vi "PRIME Telescope Convert HHMMSS string.vi"(10 "RA String":string) -> (1 "Array":dbl[](array[numeric]), 2 "Right Ascension":T1)   [LabVIEW 2024, in "PRIME Telescope.lvclass"]
uses:
  PRIME Telescope.lvclass
  library/lib cluster HH MM SEC.ctl
  <vilib>/regexp/Match Regular Expression.xnode
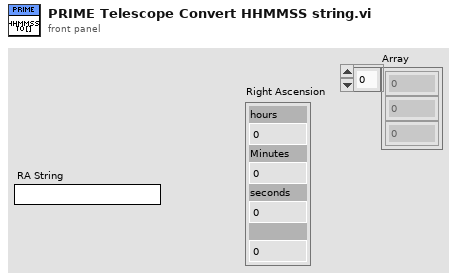
[diagram p1: front panel]
types:
  T1 = typedef "lib cluster HH MM SEC.ctl" = cluster{"hours":dbl, "Minutes":dbl, "seconds":dbl, "sign":dbl}
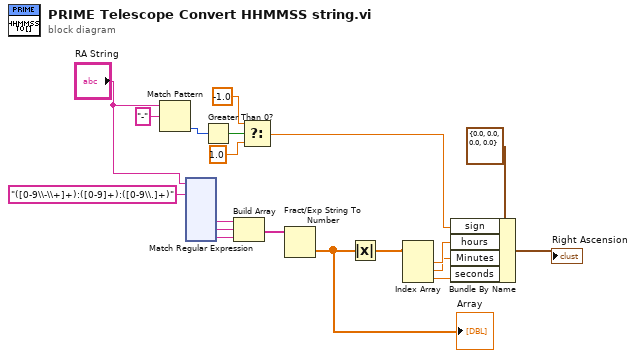
[diagram p0: block diagram]
diagram:
  n1 = Match Pattern(string="RA String", regular expression="-") -> (offset past match=w12:i32)  [unwired: 1 in, 3 out]
  n2 = xnode "Match Regular Expression"("input string"="RA String", "regular expression"="([0-9\\-\\+]+):([0-9]+):([0-9\\.]+)") -> ("submatch 1"=w18:string, "submatch 2"=w17:string, "submatch 3"=w16:string)  [unwired: 4 in, 5 out]
  n3 = Greater Than 0?(x=w12) -> (x > 0?=w4:bool)
  n4 = Build Array(w18, w17, w16) -> (w15:string[])
  n5 = Select(t=-1.0, s=w4, f=1.0) -> (s? t:f=w3:dbl)
  n6 = Fract/Exp String To Number(string=w15) -> (number=w11:dbl[])  [unwired: 3 in, 1 out]
  "Array" <- w11
  n7 = Absolute Value(x=w11) -> (abs(x)=w9:dbl[])
  n8 = Index Array(array=w9) -> (element #1=w8:dbl, element #2=w7:dbl, element #3=w6:dbl)  [unwired: 3 in]
  n9 = Bundle By Name(cluster=T1 {"hours"=0.0, "Minutes"=0.0, "seconds"=0.0, "sign"=0.0} ("Right Ascension"), "sign"=w3, "hours"=w8, "Minutes"=w7, "seconds"=w6) -> (→"Right Ascension":T1)
